vi "Modbus Slave Simulator.vi"() -> ()   [LabVIEW 2021]
doc: "A basic Modbus slave. Simulates the behavior of a PLC or other modbus device by updating input registers with changing data."
uses:
  Modbus_v121c/API/Wrapper/Create TCP Slave.vi
  Stop Global.vi
  Modbus_v121c/API/Slave/Modbus Slave.lvclass
  Modbus_v121c/API/Wrapper/API Main.lvlib
  <vilib>/ptbypt/NI_PtbyPt.lvlib
panel:
  in  "Simulation Parameters":T1(array[cluster])=[{"Input Register"=30001, "Pattern"=enum."Sine"}, {"Input Register"=30002, "Pattern"=enum."Sawtooth"}]
  # "Modbus Slave Simulator\n\nSimulates the behavior of a Modbus Slave device (PLC)."
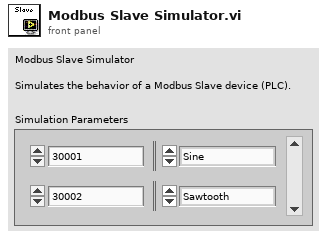
[diagram p1: front panel]
types:
  T1 = cluster{"Input Register":u16, "Pattern":enum16{"Sine", "Sawtooth", "Random"}}[]
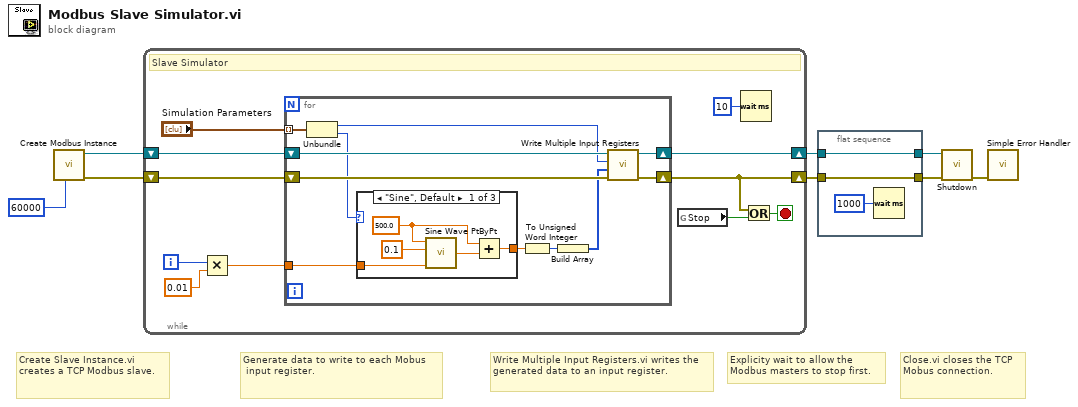
[diagram p0: block diagram]
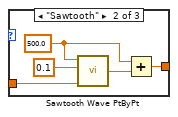
[diagram p2: hidden frame]
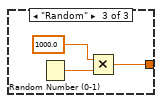
[diagram p3: hidden frame]
diagram:
  # "Explicity wait to allow the\nModbus masters to stop first."
  # "Close.vi closes the TCP\nMobus connection."
  # "Write Multiple Input Registers.vi writes the generated data to an input register."
  # "Generate data to write to each Mobus\n input register."
  # "Create Slave Instance.vi\ncreates a TCP Modbus slave."
  n1 = call-poly "Create Modbus Instance.vi"("read operation timeout"=60000) -> ("error out"=w7:errorcluster, "TCP slave instance"=w8:refnum<class "Modbus Slave.lvclass">)  [unwired: 9 in]
  n2 = while {
    shift-right: [w14] -> w5
    shift-left: w8 -> [w19]
    shift-right: [w13] -> w3
    shift-left: w7 -> [w18]
    i -> [w17]
    stop <- w12 stop-if-true
    # "Slave Simulator"
    n3 = Multiply(x=w17, y=0.01) -> (x*y=w15:dbl)
    n4 = for {
      tunnel: w15 -> [w28]
      shift-right: [w24] -> w14
      shift-left: w19 -> [w30]
      shift-right: [w23] -> w13
      shift-left: w18 -> [w29]
      tunnel: "Simulation Parameters" -> [w22] mode=indexing
      n5 = Unbundle(w22) -> ("Input Register"=w21:u16, "Pattern"=w20:enum16{"Sine", "Sawtooth", "Random"})
      n6 = case shown="\"Sine\", Default" w20 {
        tunnel: w28 -> [w32 w37 _]
        tunnel: [w31 w36 w42] -> w27
        frame "Sine", Default {
          w33 = 500.0 ("amplitude")
          n7 = call <vilib>:"Sine Wave PtByPt.vi"("time"=w32, "frequency"=0.1, "amplitude"=w33) -> ("sine wave"=w34:dbl)  [unwired: 1 in]
          n8 = Add(x=w33, y=w34) -> (x+y=w31:dbl)
        }
        frame "Sawtooth" {
          w38 = 500.0 ("amplitude")
          n9 = call <vilib>:"Sawtooth Wave PtByPt.vi"("time"=w37, "frequency"=0.1, "amplitude"=w38) -> ("sawtooth wave"=w39:dbl)  [unwired: 1 in]
          n10 = Add(x=w38, y=w39) -> (x+y=w36:dbl)
        }
        frame "Random" {
          n11 = Random Number (0-1)() -> (number: 0 to 1=w43:dbl)
          n12 = Multiply(x=1000.0, y=w43) -> (x*y=w42:dbl)
        }
      }
      n13 = To Unsigned Word Integer(number=w27) -> (unsigned 16bit integer=w26:u16)
      n14 = Build Array(w26) -> (w25:u16[])
      n15 = call-dynamic "Write Multiple Input Registers.vi"("error in (no error)"=w29, "input register values"=w25, "starting address"=w21, "Modbus slave in"=w30) -> ("error out"=w23:errorcluster, "Modbus slave out"=w24:refnum<class "Modbus Slave.lvclass">)  [unwired: 6 in]
    }
    n16 = global read "Stop Global.vi" "Stop"() -> (w10:bool)
    n17 = Wait (ms)(milliseconds to wait=u32 10) -> ()  [unwired: 1 out]
    n18 = Or(x=w13, y=w10) -> (x .or. y?=w12:bool)
  }
  n19 = flat-sequence {
    tunnel: w5 -> [w46]
    tunnel: [w46] -> w4
    tunnel: [w45] -> w2
    tunnel: w3 -> [w45]
    frame #0 {
      n20 = Wait (ms)(milliseconds to wait=u32 1000) -> ()  [unwired: 1 out]
    }
  }
  n21 = call-dynamic "Shutdown.vi"("error in (no error)"=w2, "Modbus slave in"=w4) -> ("error out"=w6:errorcluster)  [unwired: 9 in]
  n22 = call <vilib>:"Simple Error Handler.vi"("error in (no error)"=w6) -> ()  [unwired: 4 in, 5 out]
